vi "differential_derivative.vi"(10 "X":dbl[](array[numeric]), 11 "Y":dbl[](array[numeric])) -> (2 "X":dbl[](array[numeric]), 3 "dY/dX":dbl[](array[numeric]))   [LabVIEW 2017]
uses:
  <vilib>/Analysis/NI_AALPro.lvlib
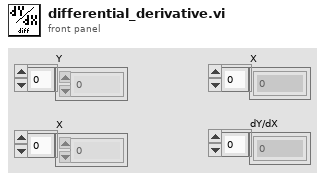
[diagram p1: front panel]
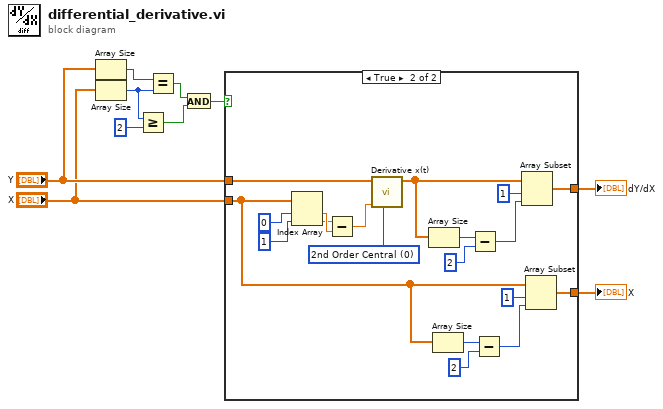
[diagram p0: block diagram]
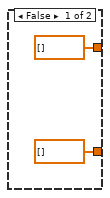
[diagram p2: hidden frame]
diagram:
  n1 = Array Size(array="Y") -> (size(s)=w6:i32)
  n2 = Array Size(array="X") -> (size(s)=w5:i32)
  n3 = Greater Or Equal?(x=w5, y=2) -> (x >= y?=w2:bool)
  n4 = Equal?(x=w6, y=w5) -> (x = y?=w3:bool)
  n5 = And(x=w3, y=w2) -> (x .and. y?=w1:bool)
  n6 = case shown="True" w1 {
    tunnel: [dbl[] [] w31] -> w10
    tunnel: [dbl[] [] w30] -> w9
    tunnel: "Y" -> [_ w14]
    tunnel: "X" -> [_ w13]
    frame False {
    }
    frame True {
      w17 = u16 0 items=["2nd Order Central", "4th Order Central", "Forward", "Backward"] ("method")
      n7 = Index Array(array=w13, index #1=0 ("index"), index #2=1 ("index")) -> (element #1=w19:dbl, element #2=w18:dbl)
      n8 = Subtract(x=w18, y=w19) -> (x-y=w20:dbl)
      n9 = call <vilib>:"Derivative x(t).vi"("method"=w17, "dt"=w20, "X"=w14) -> ("dX/dt"=w22:dbl[])  [unwired: 7 in, 1 out]
      n10 = Array Size(array=w22) -> (size(s)=w23:i32)
      n11 = Array Size(array=w13) -> (size(s)=w27:i32)
      n12 = Subtract(x=w23, y=2) -> (x-y=w25:i32)
      n13 = Subtract(x=w27, y=2) -> (x-y=w29:i32)
      n14 = Array Subset(array=w22, index=1, length=w25) -> (w30:dbl[])
      n15 = Array Subset(array=w13, index=1, length=w29) -> (w31:dbl[])
    }
  }
  "X" <- w10
  "dY/dX" <- w9
